vi "Write Log Line.vi"(10 "log line":string, 11 "string handler in":refnum<class "String Handler.lvclass">) -> (0 "error out":errorcluster, 3 "string handler out":refnum<class "String Handler.lvclass">)   [LabVIEW 2018, in "GLog.lvlib" / "String Handler.lvclass"]
uses:
  String Handler.lvclass
  String Handler.lvclass/String Handler.ctl
  <vilib>/Utility/error.llb/Trim Whitespace One-Sided.vi
panel:
  # "Connector Pane"
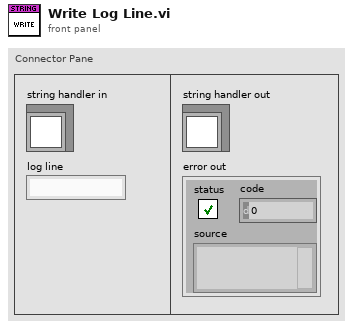
[diagram p1: front panel]
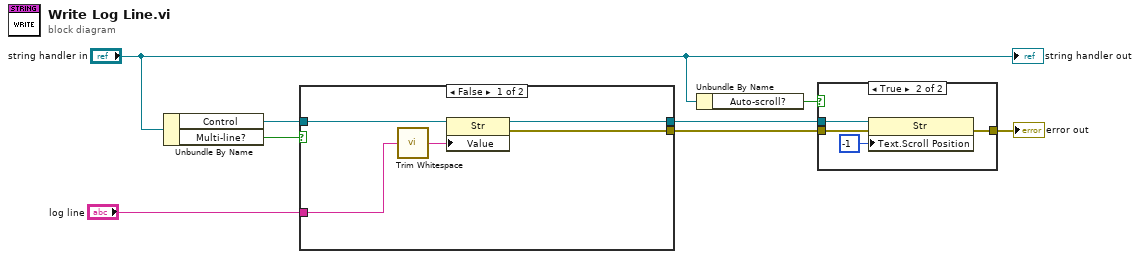
[diagram p0: block diagram]
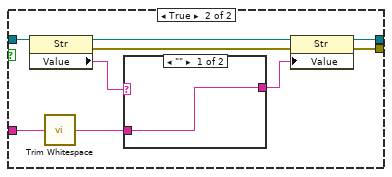
[diagram p2: hidden frame]
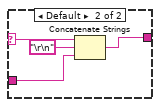
[diagram p3: hidden frame]
diagram:
  n1 = Unbundle By Name("string handler in") -> ("Control"=w8:refnum<vi>, "Multi-line?"=w6:bool)
  n2 = case shown="False" w6 {
    tunnel: w8 -> [w13 w22]
    tunnel: "log line" -> [w12 w21]
    tunnel: [w10 w17] -> w2
    tunnel: [w9 w16] -> w3
    frame False {
      n3 = call <vilib>:"Trim Whitespace.vi"("string"=w12) -> ("trimmed string"=w11:string)  [unwired: 1 in]
      n4 = property class="Str"(reference=w13, "Value"=w11) -> (reference out=w9:refnum<vi>, error out=w10:errorcluster)  [unwired: 1 in]
    }
    frame True {
      n5 = property class="Str"(reference=w22) -> (reference out=w20:refnum<vi>, error out=w18:errorcluster, "Value"=w15:string)  [unwired: 1 in]
      n6 = call <vilib>:"Trim Whitespace.vi"("string"=w21) -> ("trimmed string"=w19:string)  [unwired: 1 in]
      n7 = case shown="\"\"" w15 {
        selector: w15 -> [_ w25]
        tunnel: w19 -> [w23 w26]
        tunnel: [w23 w24] -> w14
        frame "" {
        }
        frame Default {
          n8 = Concatenate Strings(w25, "\r\n", w26) -> (w24:string)
        }
      }
      n9 = property class="Str"(reference=w20, error in=w18, "Value"=w14) -> (reference out=w16:refnum<vi>, error out=w17:errorcluster)
    }
  }
  n10 = Unbundle By Name("string handler in") -> ("Auto-scroll?"=w4:bool)
  n11 = case shown="True" w4 {
    tunnel: w3 -> [_ w32]
    tunnel: w2 -> [w28 w31]
    tunnel: [w28 w29] -> w1
    frame False {
    }
    frame True {
      n12 = property class="Str"(reference=w32, error in=w31, "Text.Scroll Position"=-1) -> (error out=w29:errorcluster)  [unwired: 1 out]
    }
  }
  "error out" <- w1
  "string handler out" <- "string handler in"
